vi "Stimulus.CreateNIVSCSVFile.vi"(8 "error in":errorcluster, 9 "Add DMM Sweep":bool, 10 "DUTs":bool[](array[boolean])=[FALSE, FALSE, FALSE, FALSE, FALSE, FALSE, FALSE, FALSE, FALSE], 11 "Path":path) -> (0 "error out":errorcluster, 3 "Saved Path":path)   [LabVIEW 2015, in "RT Sequence Creation.lvlib"]
uses:
  RT Sequence Creation.lvlib
  Shared/Shared.lvlib
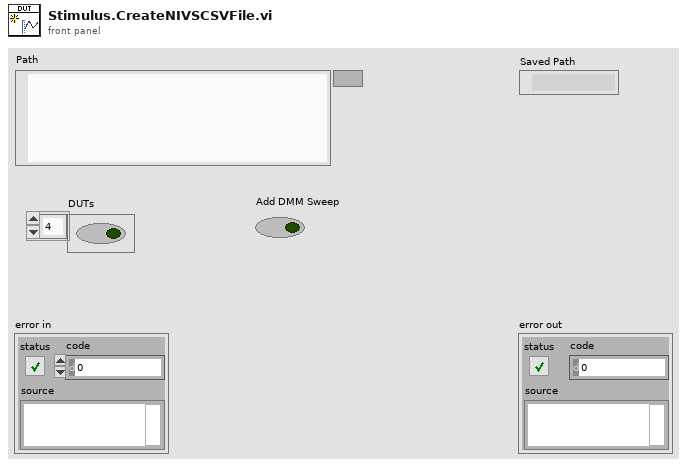
[diagram p1: front panel]
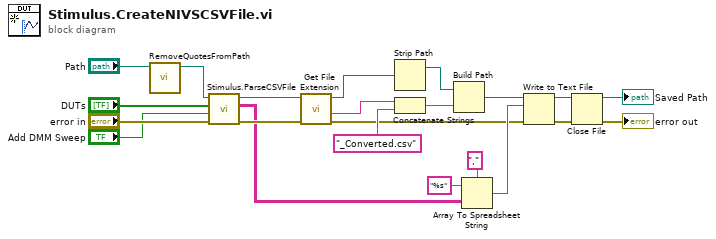
[diagram p0: block diagram]
diagram:
  n1 = call "RemoveQuotesFromPath.vi"("Data"="Path") -> ("Path"=w2:path)  [unwired: 9 in, 1 out]
  n2 = call "Stimulus.ParseCSVFile.vi"("error in (no error)"="error in", "Add DMM Sweep"="Add DMM Sweep", "DUTs"="DUTs", "Path"=w2) -> ("error out"=w13:errorcluster, "NICSVArray"=w5:string[][], "path"=w12:path)  [unwired: 5 in]
  n3 = call <vilib>:"Get File Extension.vi"("error in (no error)"=w13, "file"=w12) -> ("error out"=w11:errorcluster, "filename without extension"=w17:string, "dup file"=w19:path)  [unwired: 5 in, 2 out]
  n4 = Strip Path(path=w19) -> (stripped path=w18:path)  [unwired: 1 out]
  n5 = Concatenate Strings(w17, "_Converted.csv" ("string")) -> (w16:string)
  n6 = Build Path(base path=w18, name or relative path=w16) -> (appended path=w14:path)
  n7 = Array To Spreadsheet String(delimiter (Tab)=",", array=w5, 3:"%s" ("format string")) -> (spreadsheet string=w20:string)
  n8 = Write to Text File(file (use dialog)=w14, text=w20, error in=w11) -> (refnum out=w10:refnum<file>, error out=w9:errorcluster)  [unwired: 1 in, 1 out]
  n9 = Close File(refnum=w10, error in=w9) -> (path=→"Saved Path":path, error out=→"error out":errorcluster)
